vi "UPDATE VI.vi"(9 "Array":string[](array[string]), 10 "columns":string[](array[string]), 11 "TABELLA":string) -> (3 "String":string)   [LabVIEW 2019]
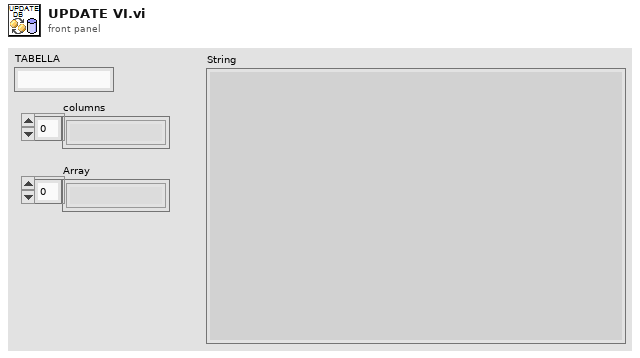
[diagram p1: front panel]
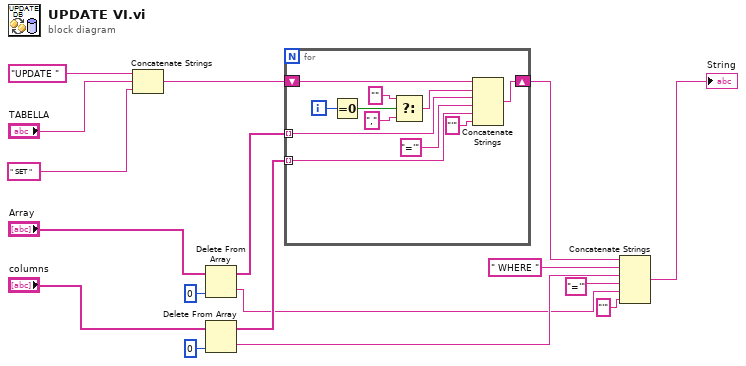
[diagram p0: block diagram]
diagram:
  n1 = Concatenate Strings("UPDATE ", "TABELLA", " SET " ("string")) -> (w17:string)
  n2 = Delete From Array(array="Array", index=0) -> (deleted portion=w3:string, array with subset deleted=w8:string[])  [unwired: 1 in]
  n3 = Delete From Array(array="columns", index=0) -> (deleted portion=w5:string, array with subset deleted=w6:string[])  [unwired: 1 in]
  n4 = for {
    tunnel: w8 -> [w28] mode=indexing
    shift-right: [w21] -> w13
    shift-left: w17 -> [w23]
    tunnel: w6 -> [w19] mode=indexing
    i -> [w27]
    n5 = Equal To 0?(x=w27) -> (x = 0?=w26:bool)
    n6 = Select(t="" ("String"), s=w26, f=",") -> (s? t:f=w22:string)
    n7 = Concatenate Strings(w23, w22, w28, "='" ("string"), w19, "'" ("string")) -> (w21:string)
  }
  n8 = Concatenate Strings(w13, " WHERE " ("string"), w5, "='" ("string"), w3, "'" ("string")) -> (→"String":string)
